vi "Sub03_03_ReadPosTxt.vi"(8 "error in (no error)":errorcluster, 11 "appended path":path) -> (0 "error out":errorcluster, 3 "output cluster":T1)   [LabVIEW 2019]
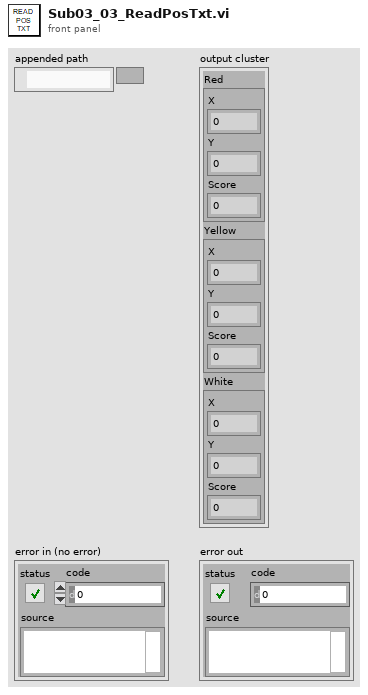
[diagram p1: front panel]
types:
  T1 = cluster{"Red":cluster{"X":u32, "Y":u32, "Score":u32}, "Yellow":cluster{"X":u32, "Y":u32, "Score":u32}, "White":cluster{"X":u32, "Y":u32, "Score":u32}}
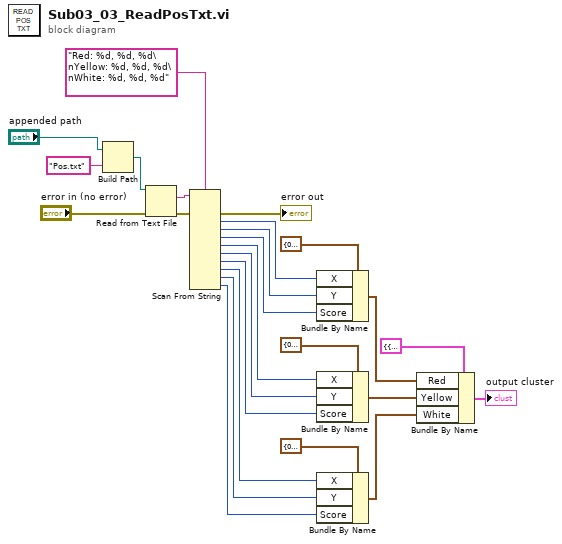
[diagram p0: block diagram]
diagram:
  n1 = Build Path(base path="appended path", name or relative path="Pos.txt") -> (appended path=w3:path)
  n2 = Read from Text File(file (use dialog)=w3, error in="error in (no error)") -> (text=w5:string, error out=w6:errorcluster)  [unwired: 2 in, 2 out]
  n3 = Scan From String(format string="Red: %d, %d, %d\nYellow: %d, %d, %d\nWhite: %d, %d, %d", input string=w5, error in=w6) -> (error out=→"error out":errorcluster, output 1=w7:i32, output 2=w8:i32, output 3=w9:i32, output 4=w10:i32, output 5=w11:i32, output 6=w12:i32, output 7=w14:i32, output 8=w15:i32, output 9=w16:i32)  [unwired: 10 in, 2 out]
  n4 = Bundle By Name(cluster=cluster{"X":u32, "Y":u32, "Score":u32} {"X"=0, "Y"=0, "Score"=0} ("Cluster"), "X"=w7, "Y"=w8, "Score"=w9) -> (w18:cluster{"X":u32, "Y":u32, "Score":u32})
  n5 = Bundle By Name(cluster=cluster{"X":u32, "Y":u32, "Score":u32} {"X"=0, "Y"=0, "Score"=0} ("Cluster"), "X"=w10, "Y"=w11, "Score"=w12) -> (w19:cluster{"X":u32, "Y":u32, "Score":u32})
  n6 = Bundle By Name(cluster=cluster{"X":u32, "Y":u32, "Score":u32} {"X"=0, "Y"=0, "Score"=0} ("Cluster"), "X"=w14, "Y"=w15, "Score"=w16) -> (w20:cluster{"X":u32, "Y":u32, "Score":u32})
  n7 = Bundle By Name(cluster=T1 {"Red"={"X"=0, "Y"=0, "Score"=0}, "Yellow"={"X"=0, "Y"=0, "Score"=0}, "White"={"X"=0, "Y"=0, "Score"=0}} ("output cluster"), "Red"=w18, "Yellow"=w19, "White"=w20) -> (→"output cluster":T1)
